vi "H5Tcommit_anon.vi"(5 "Datatype Access Property List":T1, 7 "Datatype Creation Property List":T1, 8 "error in (no error)":errorcluster, 9 "HDF5 Type Ref":T1, 11 "HDF5 Location Ref":T1) -> (0 "error out":errorcluster, 3 "HDF5 Location Ref out":T1)   [LabVIEW 2017]
doc: "Commits a transient datatype to a file, creating a new named datatype, \n but does not link it into the file structure."
uses:
  <vilib>/UPVI/lvhdf5/library.llb/HDF5 Ref.ctl
  <vilib>/UPVI/lvhdf5/hdf5.dll
panel:
  # "LVHDF5 Toolkit\nCopyright (c) 2005-2013 by Jason D. Sommerville\nCopyright (c) 2014 by UPVI, LLC.\n\nThis use and distribution of this file is governed by the terms found in \nLICENSE.txt distributed with this toolkit and installed at\n <user.lib>\\_lvhdf5\\LICENSE.txt"
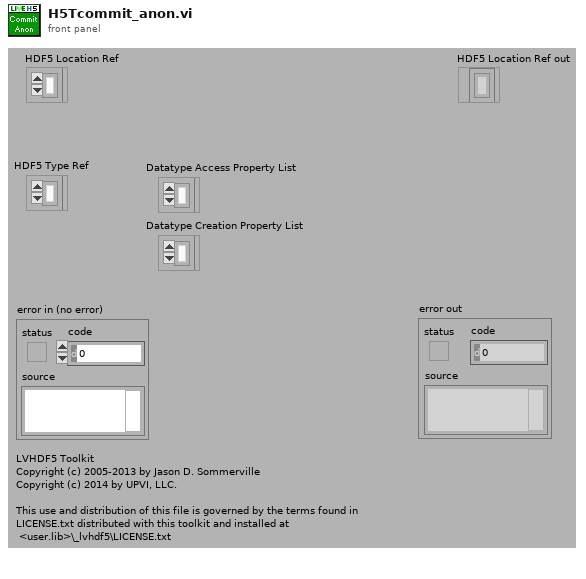
[diagram p1: front panel]
types:
  T1 = typedef "HDF5 Ref.ctl" = refnum<k1>
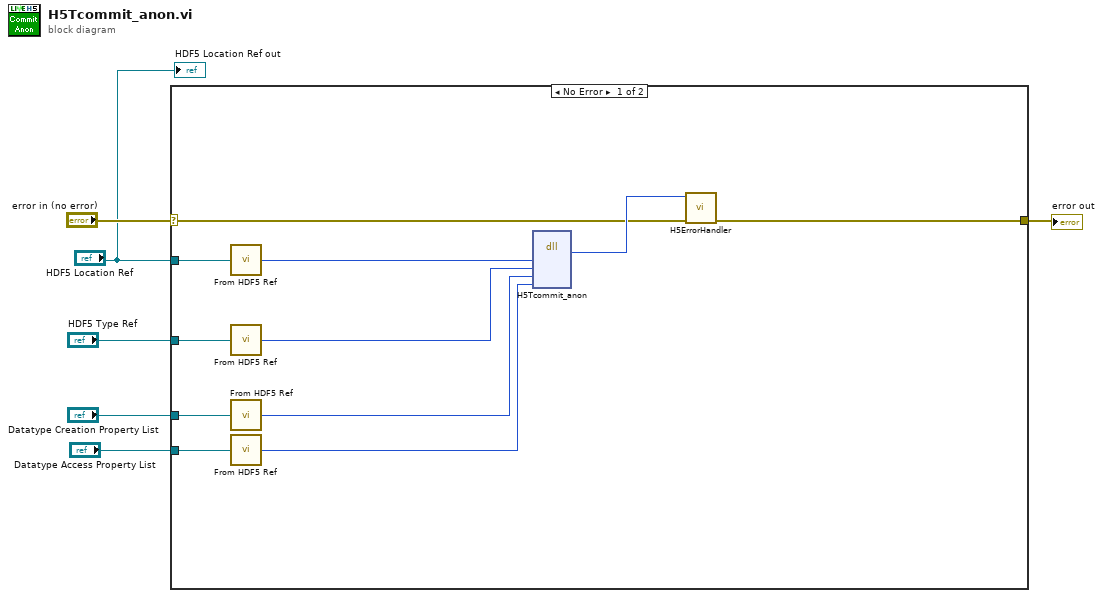
[diagram p0: block diagram]
diagram:
  n1 = case shown="No Error" "error in (no error)" {
    selector: "error in (no error)" -> [w15 w18]
    tunnel: [w14 w18] -> w5
    tunnel: "HDF5 Location Ref" -> [w17 _]
    tunnel: "HDF5 Type Ref" -> [w12 _]
    tunnel: "Datatype Creation Property List" -> [w10 _]
    tunnel: "Datatype Access Property List" -> [w9 _]
    frame No Error {
      n2 = call <vilib>:"From HDF5 Ref.vi"("HDF5 Ref"=w17) -> ("I32"=w13:i32)
      n3 = call <vilib>:"From HDF5 Ref.vi"("HDF5 Ref"=w12) -> ("I32"=w11:i32)
      n4 = call <vilib>:"From HDF5 Ref.vi"("HDF5 Ref"=w10) -> ("I32"=w8:i32)
      n5 = call <vilib>:"From HDF5 Ref.vi"("HDF5 Ref"=w9) -> ("I32"=w7:i32)
      n6 = dll-call lib="C:/Program Files/National Instruments/LabVIEW 2017/vi.lib/UPVI/lvhdf5/hdf5.dll" fn="H5Tcommit_anon"("loc_id"=w13, "dtype_id"=w11, "tcpl_id"=w8, "tapl_id"=w7) -> ("return type"=w16:i32)  [unwired: 7 in, 2 out]
      n7 = call <vilib>:"H5ErrorHandler.vi"("error in (no error)"=w15, "herr_t"=w16) -> ("error out"=w14:errorcluster)  [unwired: 3 in, 4 out]
    }
    frame Error {
    }
  }
  "error out" <- w5
  "HDF5 Location Ref out" <- "HDF5 Location Ref"
